vi "PH_Beckhoff-16BB.ProcCases.vi"(0 "i ref in":refnum<vi>, 1 "selector":string, 2 "Data":T1, 3 "call cluster":T2={"Object"="", "Selector"="", "CallType"=enum."synchronous", "Async Object"="", "Async Selector"="", "Data Descriptor"="", "Data"=[], "Error #"=0, "Expire"=0}, 5 "error in (no error)":errorcluster) -> (14 "i ref out":refnum<vi>, 17 "answer cluster":T2={"Object"="", "Selector"="", "CallType"=enum."synchronous", "Async Object"="", "Async Selector"="", "Data Descriptor"="", "Data"=[], "Error #"=0, "Expire"=0}, 19 "error out":errorcluster)   [LabVIEW 2014, in "PH_Beckhoff-16BB.lvlib"]
doc: "This method is called by a process from within the default case in the event loop. The methods of a class that are linked to events will be called from THIS method. Add your code here."
uses:
  PH_Beckhoff-16BB.lvlib
  CS_Core/CSSystem/CoreDefs/CoreDefs.call_type.ctl
  CS_Core/BaseProcess/BaseProcess.descriptor string definition.ctl
  CS_Core/CSSystem/CoreDefs/CoreDefs.rawDataType.ctl
  PH_Basics/PH_PSDBWriter/PH_PSDBWriter.Thread Commands.ctl
  CS_Core/CSSystem/CoreLib/CoreLib.string 2 byte array.vi
  PH_Beckhoff/PH_Beckhoff.lvlib
  CS_Core/CSSystem/CoreLib/CoreLib.lvlib
  CS_Core/BaseProcess/BaseProcess.lvlib
  CS_Core/CAEObj/CAEObj.lvlib
  PH_Basics/PH_PSDBWriter/PH_PSDBWriter.lvlib
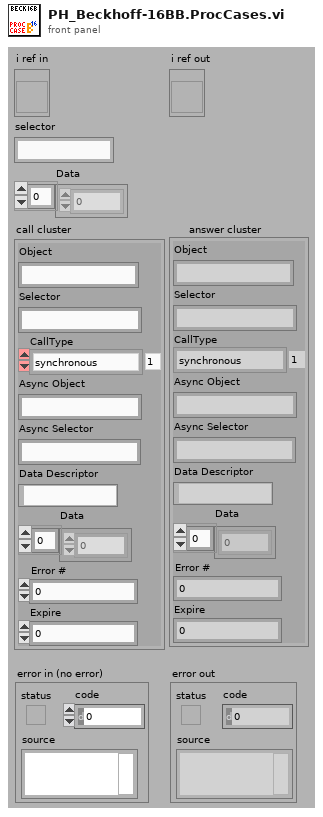
[diagram p1: front panel]
types:
  T1 = typedef "CoreDefs.rawDataType.ctl" = i8[]
  T2 = typedef "CoreDefs.call_type.ctl" = cluster{"Object":string, "Selector":string, "CallType":enum16{"simple", "synchronous", "asynchronous"}, "Async Object":string, "Async Selector":string, "Data Descriptor":T3, "Data":T1, "Error #":i32, "Expire":u32}
  T3 = typedef "BaseProcess.lvlib/BaseProcess.descriptor string definition.ctl" = string
  T4 = typedef "PH_Beckhoff-16BB.lvlib/PH_Beckhoff-16BB.i attribute.ctl" = cluster{"PA Chiller":cluster{"PSDB":cluster{"Status Service ID":i32, "Instance ID":i32, "Data Status":T5, "Ref Status":refnum<vi>, "Error Code":i32}, "Status":cluster{"GUI Ref":refnum<vi>, "Status Service ID":i32, "Status":T6}, "DIs":cluster{"Flow Control":cluster{"GUI Ref":refnum<vi>, "# in Data":i32}, "High-Temp":cluster{"GUI Ref":refnum<vi>, "# in Data":i32}, "Conductivity":cluster{"GUI Ref":refnum<vi>, "# in Data":i32}, "Niveau":cluster{"GUI Ref":refnum<vi>, "# in Data":i32}}, "PSDB Thread":cluster{"Ref":refnum<vi>, "Q-Ref":refnum<queue>}}, "PSDB":cluster{"Shot #":i32, "Subsystem":T7}, "Racktype":string, "PSDB Credentials":T8}
  T5 = typedef "PH_PSDBWriter.lvlib/PH_PSDBWriter.Data Status.ctl" = i16
  T6 = typedef "PH_StatusHandler.lvlib/PH_StatusHandler.Status.ctl" = i16
  T7 = typedef "PH_PSDBWriter.lvlib/PH_PSDBWriter.PHELIX-Subsystems.ctl" = i32
  T8 = typedef "PH_Common.lvlib/PH_Connection.PSDB Credentials.ctl" = cluster{"PW":string, "ID":string, "DS":string}
  T9 = typedef "PH_PSDBWriter.lvlib/PH_PSDBWriter.Thread Commands.ctl" = u16
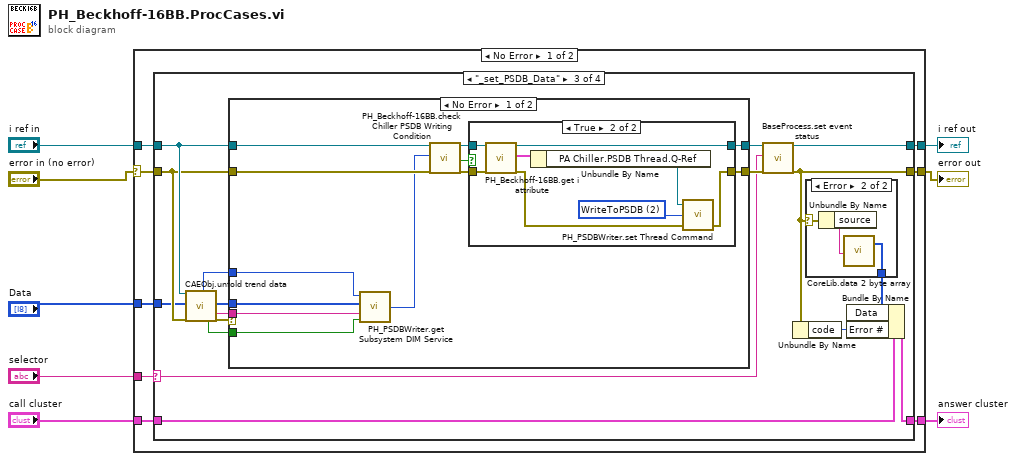
[diagram p0: block diagram]
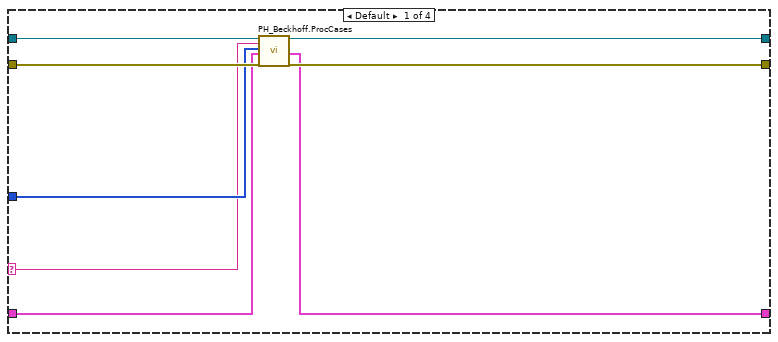
[diagram p2: hidden frame]
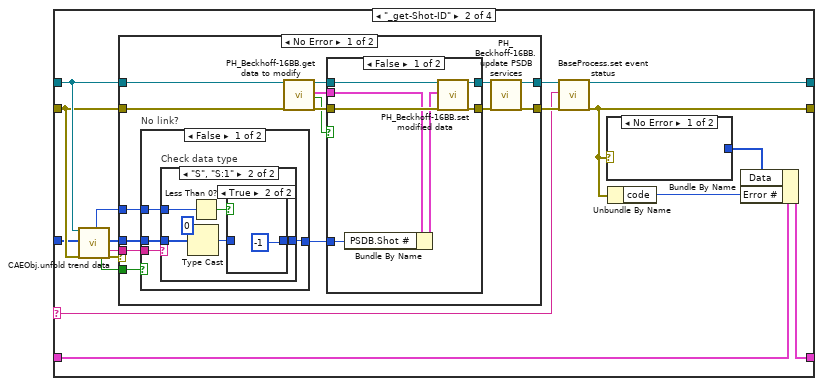
[diagram p3: hidden frame]
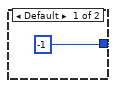
[diagram p5: hidden frame]
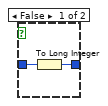
[diagram p6: hidden frame]
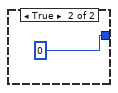
[diagram p7: hidden frame]
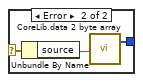
[diagram p9: hidden frame]
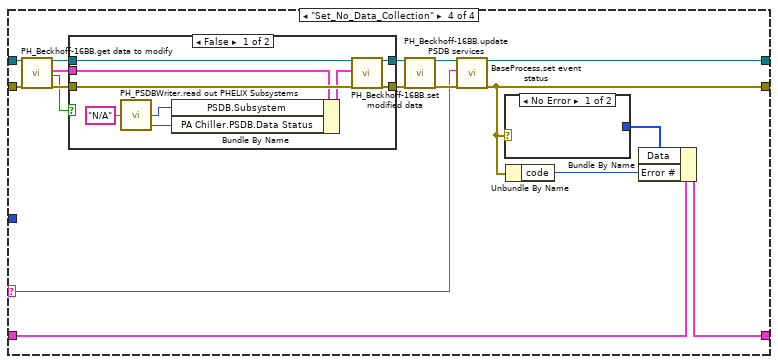
[diagram p13: hidden frame]
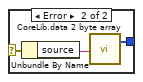
[diagram p15: hidden frame]
diagram:
  n1 = case shown="No Error" "error in (no error)" {
    selector: "error in (no error)" -> [w9 w161]
    tunnel: "selector" -> [w16 _]
    tunnel: [w15 w162] -> w7
    tunnel: "Data" -> [w14 _]
    tunnel: "call cluster" -> [w13 w162]
    tunnel: "i ref in" -> [w12 w163]
    tunnel: [w11 w163] -> w3
    tunnel: [w10 w161] -> w2
    frame No Error {
      n2 = case shown="\"_set_PSDB_Data\"" w16 {
        selector: w16 -> [w18 w26 w87 w136]
        tunnel: w14 -> [w19 w25 w86 _]
        tunnel: w12 -> [w17 w32 w93 w142]
        tunnel: [w24 w30 w91 w140] -> w11
        tunnel: w13 -> [w20 w28 w89 w138]
        tunnel: [w21 w27 w88 w137] -> w15
        tunnel: w9 -> [w23 w31 w92 w141]
        tunnel: [w22 w29 w90 w139] -> w10
        frame Default {
          n3 = call "PH_Beckhoff.ProcCases.vi"("i ref in"=w17, "selector"=w18, "Data"=w19, "call cluster"=w20, "error in (no error)"=w23) -> ("i ref out"=w24:refnum<vi>, "answer cluster"=w21:T2, "error out"=w22:errorcluster)  [unwired: 12 in]
        }
        frame "_get-Shot-ID" {
          n4 = call "CAEObj.unfold trend data.vi"("i ref in"=w32, "raw trend data"=w25, "error in (no error)"=w31) -> ("quality"=w37:i32, "no link"=w35:bool, "data"=w40:i8[], "typeDescriptor"=w41:string, "error out"=w36:errorcluster)  [unwired: 8 in, 4 out]
          n5 = case shown="No Error" w36 {
            tunnel: w31 -> [w52 w82]
            tunnel: [w45 w81] -> w38
            tunnel: [w43 w82] -> w39
            tunnel: w32 -> [w51 w81]
            tunnel: w35 -> [w56 _]
            tunnel: w41 -> [w55 _]
            tunnel: w40 -> [w54 _]
            tunnel: w37 -> [w53 _]
            frame No Error {
              n6 = case "No link?" shown="False" w56 {
                tunnel: [w69 0] -> w46
                tunnel: w53 -> [w68 _]
                tunnel: w54 -> [w67 _]
                tunnel: w55 -> [w66 _]
                frame False {
                  n7 = case "Check data type" shown="\"S\", \"S:1\"" w66 {
                    tunnel: [-1 w76] -> w69
                    tunnel: w68 -> [_ w74]
                    tunnel: w67 -> [_ w72]
                    frame Default {
                    }
                    frame "S", "S:1" {
                      n8 = Type Cast(type=i16 0, x=w72) -> (*(type *) &x=w71:i16)
                      n9 = Less Than 0?(x=w74) -> (x < 0?=w75:bool)
                      n10 = case shown="True" w75 {
                        tunnel: [w77 -1] -> w76
                        tunnel: w71 -> [w78 _]
                        frame False {
                          n11 = To Long Integer(number=w78) -> (32bit integer=w77:i32)
                        }
                        frame True {
                        }
                      }
                    }
                  }
                }
                frame True {
                }
              }
              n12 = call "PH_Beckhoff-16BB.get data to modify.vi"("i ref in"=w51, "error in (no error)"=w52) -> ("i ref out"=w49:refnum<vi>, "i attribute"=w47:T4, "timed out"=w48:bool, "error out"=w50:errorcluster)  [unwired: 14 in]
              n13 = case shown="False" w48 {
                tunnel: w50 -> [w63 w64]
                tunnel: [w62 w64] -> w42
                tunnel: w49 -> [w61 w65]
                tunnel: [w60 w65] -> w44
                tunnel: w47 -> [w59 _]
                tunnel: w46 -> [w57 _]
                frame False {
                  n14 = Bundle By Name(cluster=w59, "PSDB.Shot #"=w57) -> (w58:T4)
                  n15 = call "PH_Beckhoff-16BB.set modified data.vi"("i ref in"=w61, "i attribute"=w58, "error in (no error)"=w63) -> ("i ref out"=w60:refnum<vi>, "error out"=w62:errorcluster)  [unwired: 15 in]
                }
                frame True {
                }
              }
              n16 = call "PH_Beckhoff-16BB.update PSDB services.vi"("i ref in"=w44, "error in"=w42) -> ("i ref out"=w45:refnum<vi>, "error out"=w43:errorcluster)  [unwired: 16 in]
            }
            frame Error {
            }
          }
          n17 = call "BaseProcess.set event status.vi"("i ref in"=w38, "EventStatus"=w26, "error in (no error)"=w39) -> ("i ref out"=w30:refnum<vi>, "error out"=w29:errorcluster)  [unwired: 14 in, 1 out]
          n18 = case shown="No Error" w29 {
            selector: w29 -> [_ w85]
            tunnel: [_ w83] -> w34
            frame No Error {
            }
            frame Error {
              n19 = Unbundle By Name(w85) -> ("source"=w84:string)
              n20 = call-poly "CoreLib.data 2 byte array.vi"("string"=w84) -> ("byteArray out"=w83:T1)  [unwired: 18 in]
            }
          }
          n21 = Unbundle By Name(w29) -> ("code"=w33:i32)
          n22 = Bundle By Name(cluster=w28, "Data"=w34, "Error #"=w33) -> (w27:T2)
        }
        frame "_set_PSDB_Data" {
          n23 = call "CAEObj.unfold trend data.vi"("i ref in"=w93, "raw trend data"=w86, "error in (no error)"=w92) -> ("quality"=w98:i32, "no link"=w96:bool, "data"=w101:i8[], "typeDescriptor"=w102:string, "error out"=w97:errorcluster)  [unwired: 8 in, 4 out]
          n24 = case shown="No Error" w97 {
            tunnel: w92 -> [w114 w126]
            tunnel: [w109 w125] -> w99
            tunnel: [w108 w126] -> w100
            tunnel: w93 -> [w112 w125]
            tunnel: w96 -> [w103 _]
            tunnel: w102 -> [w105 _]
            tunnel: w101 -> [w106 _]
            tunnel: w98 -> [w104 _]
            frame No Error {
              n25 = call "PH_PSDBWriter.get Subsystem DIM Service.vi"("no link"=w103, "typeDescriptor"=w105, "data"=w106, "quality"=w104) -> ("PHELIX Subsystems"=w107:T7)
              n26 = call "PH_Beckhoff-16BB.check Chiller PSDB Writing Condition.vi"("i ref in"=w112, "wanted Subsystem"=w107, "error IO"=w114) -> ("i ref out"=w110:refnum<vi>, "write Chiller Data to PSDB?"=w111:bool, "error out"=w113:errorcluster)  [unwired: 14 in]
              n27 = case shown="True" w111 {
                tunnel: w113 -> [w116 w124]
                tunnel: [w116 w120] -> w108
                tunnel: w110 -> [w115 w122]
                tunnel: [w115 w121] -> w109
                frame False {
                }
                frame True {
                  w117 = T9 2 items=["None", "GetInstanceID", "WriteToPSDB"] ("PSDB Thread Command")
                  n28 = call "PH_Beckhoff-16BB.get i attribute.vi"("i ref in"=w122, "error in (no error)"=w124) -> ("i ref out"=w121:refnum<vi>, "i attribute"=w119:T4, "error out"=w123:errorcluster)  [unwired: 15 in]
                  n29 = Unbundle By Name(w119) -> ("PA Chiller.PSDB Thread.Q-Ref"=w118:refnum<queue>)
                  n30 = call "PH_PSDBWriter.set Thread Command.vi"("error in (no error)"=w123, "PSDB Thread Command"=w117, "Queue in"=w118) -> ("error out"=w120:errorcluster)  [unwired: 2 in]
                }
              }
            }
            frame Error {
            }
          }
          n31 = call "BaseProcess.set event status.vi"("i ref in"=w99, "EventStatus"=w87, "error in (no error)"=w100) -> ("i ref out"=w91:refnum<vi>, "error out"=w90:errorcluster)  [unwired: 14 in, 1 out]
          n32 = Unbundle By Name(w90) -> ("code"=w94:i32)
          n33 = case shown="Error" w90 {
            selector: w90 -> [_ w129]
            tunnel: [_ w127] -> w95
            frame No Error {
            }
            frame Error {
              n34 = Unbundle By Name(w129) -> ("source"=w128:string)
              n35 = call-poly "CoreLib.data 2 byte array.vi"("string"=w128) -> ("byteArray out"=w127:T1)  [unwired: 18 in]
            }
          }
          n36 = Bundle By Name(cluster=w89, "Data"=w95, "Error #"=w94) -> (w88:T2)
        }
        frame "Set_No_Data_Collection" {
          n37 = call "PH_Beckhoff-16BB.get data to modify.vi"("i ref in"=w142, "error in (no error)"=w141) -> ("i ref out"=w134:refnum<vi>, "i attribute"=w132:T4, "timed out"=w133:bool, "error out"=w135:errorcluster)  [unwired: 14 in]
          n38 = case shown="False" w133 {
            tunnel: w135 -> [w155 w156]
            tunnel: [w154 w156] -> w130
            tunnel: w134 -> [w153 w157]
            tunnel: [w152 w157] -> w131
            tunnel: w132 -> [w151 _]
            frame False {
              n39 = call "PH_PSDBWriter.read out PHELIX Subsystems.vi"("Config DB Subsystem"="N/A") -> ("Metadata.Data Status"=w147:T5, "Metadata.Subsystem"=w148:T7)  [unwired: 2 in, 1 out]
              n40 = Bundle By Name(cluster=w151, "PSDB.Subsystem"=w148, "PA Chiller.PSDB.Data Status"=w147) -> (w150:T4)
              n41 = call "PH_Beckhoff-16BB.set modified data.vi"("i ref in"=w153, "i attribute"=w150, "error in (no error)"=w155) -> ("i ref out"=w152:refnum<vi>, "error out"=w154:errorcluster)  [unwired: 15 in]
            }
            frame True {
            }
          }
          n42 = call "PH_Beckhoff-16BB.update PSDB services.vi"("i ref in"=w131, "error in"=w130) -> ("i ref out"=w145:refnum<vi>, "error out"=w146:errorcluster)  [unwired: 16 in]
          n43 = call "BaseProcess.set event status.vi"("i ref in"=w145, "EventStatus"=w136, "error in (no error)"=w146) -> ("i ref out"=w140:refnum<vi>, "error out"=w139:errorcluster)  [unwired: 14 in, 1 out]
          n44 = case shown="No Error" w139 {
            selector: w139 -> [_ w160]
            tunnel: [_ w158] -> w144
            frame No Error {
            }
            frame Error {
              n45 = Unbundle By Name(w160) -> ("source"=w159:string)
              n46 = call-poly "CoreLib.data 2 byte array.vi"("string"=w159) -> ("byteArray out"=w158:T1)  [unwired: 18 in]
            }
          }
          n47 = Unbundle By Name(w139) -> ("code"=w143:i32)
          n48 = Bundle By Name(cluster=w138, "Data"=w144, "Error #"=w143) -> (w137:T2)
        }
      }
    }
    frame Error {
    }
  }
  "answer cluster" <- w7
  "i ref out" <- w3
  "error out" <- w2
